vi "Preview Single D.vi"(8 "Error In":errorcluster, 10 "index":i32, 11 "Queue in":refnum<queue>) -> (0 "Error Out":errorcluster, 1 "D Array":i16[](array[numeric]), 2 "D value":i16, 3 "SEQ out":refnum<queue>)   [LabVIEW 2019, in "FX5U SLMP Binary.lvlib"]
uses:
  FX5U SLMP Binary.lvlib
  Data Cluster.ctl
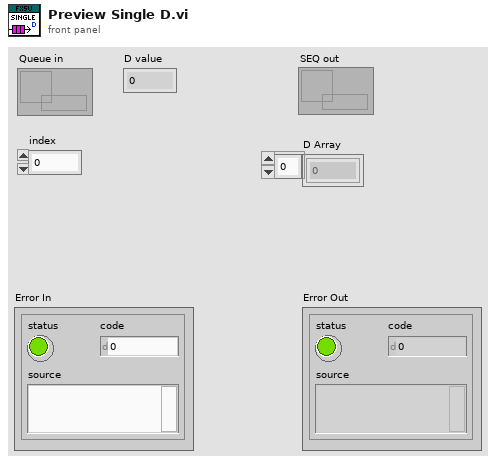
[diagram p1: front panel]
types:
  T1 = typedef "FX5U SLMP Binary.lvlib/Data Cluster.ctl" = cluster{"M Array":bool[], "D Array":i16[]}
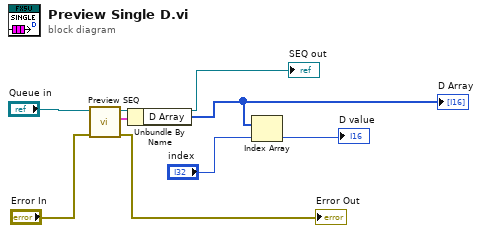
[diagram p0: block diagram]
diagram:
  n1 = call "Preview SEQ.vi"("Error In"="Error In", "SEQ in"="Queue in") -> ("Error Out"=→"Error Out":errorcluster, "Data Cluster"=w4:T1, "SEQ out"=→"SEQ out":refnum<queue>)  [unwired: 7 in]
  n2 = Unbundle By Name(w4) -> ("D Array"=w5:i16[])
  "D Array" <- w5
  n3 = Index Array(array=w5, index="index") -> (element=→"D value":i16)
